vi "AutonWait.vi"(9 "Target Time (s)":dbl, 11 "First Time?":bool) -> (1 "ElapsedTime":dbl, 3 "Completed":bool)   [LabVIEW 2016]
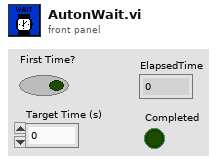
[diagram p1: front panel]
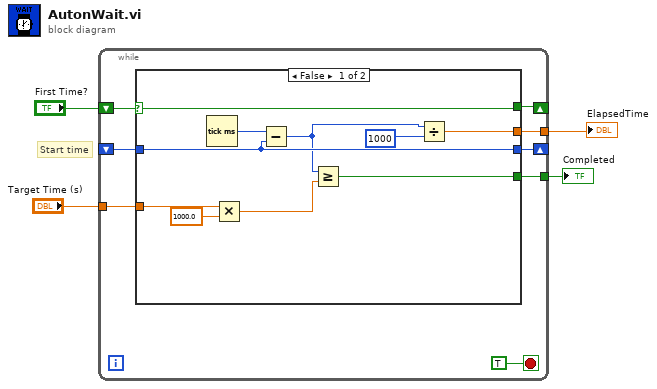
[diagram p0: block diagram]
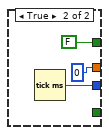
[diagram p2: hidden frame]
diagram:
  # "Start time"
  n1 = while {
    shift-right: [w10] -> _
    shift-left: "First Time?" -> [w11]
    shift-right: [w9] -> _
    shift-left: _ -> [w8]
    tunnel: "Target Time (s)" -> [w7]
    tunnel: [w6] -> w2
    tunnel: [w5] -> w1
    stop <- TRUE stop-if-true
    n2 = case shown="False" w11 {
      selector: w11 -> [w22 _]
      tunnel: [w22 FALSE] -> w10
      tunnel: [w20 w24] -> w9
      tunnel: w8 -> [w20 _]
      tunnel: w7 -> [w19 _]
      tunnel: [w16 _] -> w6
      tunnel: [w15 u32 0] -> w5
      frame False {
        n3 = Tick Count (ms)() -> (millisecond timer value=w21:u32)
        n4 = Multiply(x=w19, y=1000.0) -> (x*y=w17:dbl)
        n5 = Subtract(x=w21, y=w20) -> (x-y=w13:u32)
        n6 = Greater Or Equal?(x=w13, y=w17) -> (x >= y?=w16:bool)
        n7 = Divide(x=w13, y=u32 1000 ("x")) -> (x/y=w15:dbl)
      }
      frame True {
        n8 = Tick Count (ms)() -> (millisecond timer value=w24:u32)
      }
    }
  }
  "Completed" <- w2
  "ElapsedTime" <- w1
